vi "XY Graph to an XY Chart.vi"(8 "Chart History (10,000)":i32=10000, 9 "Clear Graph?":bool, 10 "Y Value":dbl format="%#_13g", 11 "X Value":dbl format="%#_13g") -> (0 "XY Graph":cluster{dbl[], dbl[]})   [LabVIEW 2017]
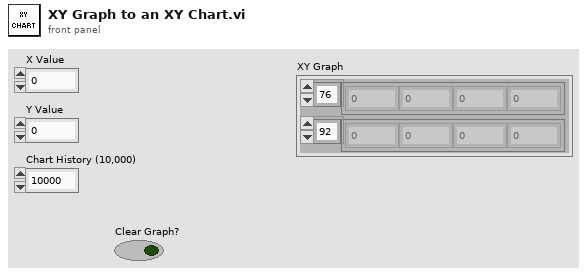
[diagram p1: front panel]
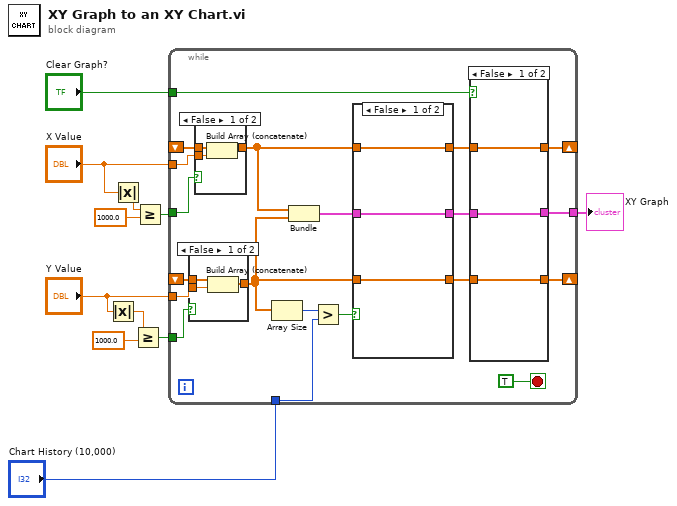
[diagram p0: block diagram]
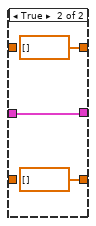
[diagram p4: hidden frame]
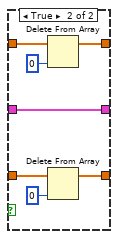
[diagram p5: hidden frame]
diagram:
  n1 = Absolute Value(x="Y Value") -> (abs(x)=w2:dbl)
  n2 = Absolute Value(x="X Value") -> (abs(x)=w5:dbl)
  n3 = Greater Or Equal?(x=w2, y=1000.0) -> (x >= y?=w1:bool)
  n4 = Greater Or Equal?(x=w5, y=1000.0) -> (x >= y?=w6:bool)
  n5 = while {
    tunnel: "X Value" -> [w31]
    tunnel: "Y Value" -> [w29]
    shift-right: [w18] -> _
    shift-left: _ -> [w30]
    shift-right: [w21] -> _
    shift-left: _ -> [w28]
    tunnel: "Chart History (10,000)" -> [w26]
    tunnel: [w16] -> w10
    tunnel: "Clear Graph?" -> [w14]
    tunnel: w6 -> [w13]
    tunnel: w1 -> [w12]
    stop <- TRUE stop-if-true
    n6 = case shown="False" w12 {
      tunnel: w29 -> [w34 _]
      tunnel: w28 -> [w33 w35]
      tunnel: [w32 w35] -> w23
      frame False {
        n7 = Build Array (concatenate)(w33, w34) -> (w32:dbl[])
      }
      frame True {
      }
    }
    n8 = case shown="False" w13 {
      tunnel: w31 -> [w38 _]
      tunnel: w30 -> [w37 w39]
      tunnel: [w36 w39] -> w20
      frame False {
        n9 = Build Array (concatenate)(w37, w38) -> (w36:dbl[])
      }
      frame True {
      }
    }
    n10 = Array Size(array=w23) -> (size(s)=w27:i32)
    n11 = Bundle(w20, w23) -> (w24:cluster{dbl[], dbl[]})  [unwired: 1 in]
    n12 = Greater?(x=w27, y=w26) -> (0:w25:bool)
    n13 = case shown="False" w25 {
      tunnel: w24 -> [w46 w49]
      tunnel: w23 -> [w48 w51]
      tunnel: [w48 w50] -> w22
      tunnel: [w47 w54] -> w19
      tunnel: w20 -> [w47 w55]
      tunnel: [w46 w49] -> w17
      frame False {
      }
      frame True {
        n14 = Delete From Array(array=w55, index=0) -> (array with subset deleted=w54:dbl[])  [unwired: 1 in, 1 out]
        n15 = Delete From Array(array=w51, index=0) -> (array with subset deleted=w50:dbl[])  [unwired: 1 in, 1 out]
      }
    }
    n16 = case shown="False" w14 {
      tunnel: w22 -> [w42 _]
      tunnel: [w42 dbl[] []] -> w21
      tunnel: w19 -> [w41 _]
      tunnel: [w41 dbl[] []] -> w18
      tunnel: [w40 w43] -> w16
      tunnel: w17 -> [w40 w43]
      frame False {
      }
      frame True {
      }
    }
  }
  "XY Graph" <- w10
